vi "Build Help.vi"(8 "Error In":errorcluster) -> (0 "Error Out":errorcluster, 3 "stdout":string)   [LabVIEW 2017, in "Scripts.lvlib"]
uses:
  Scripts.lvlib
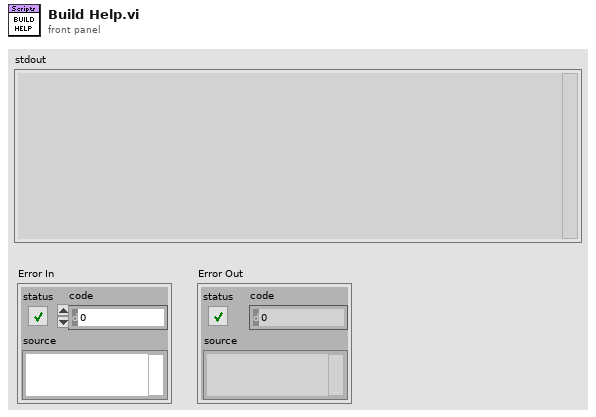
[diagram p1: front panel]
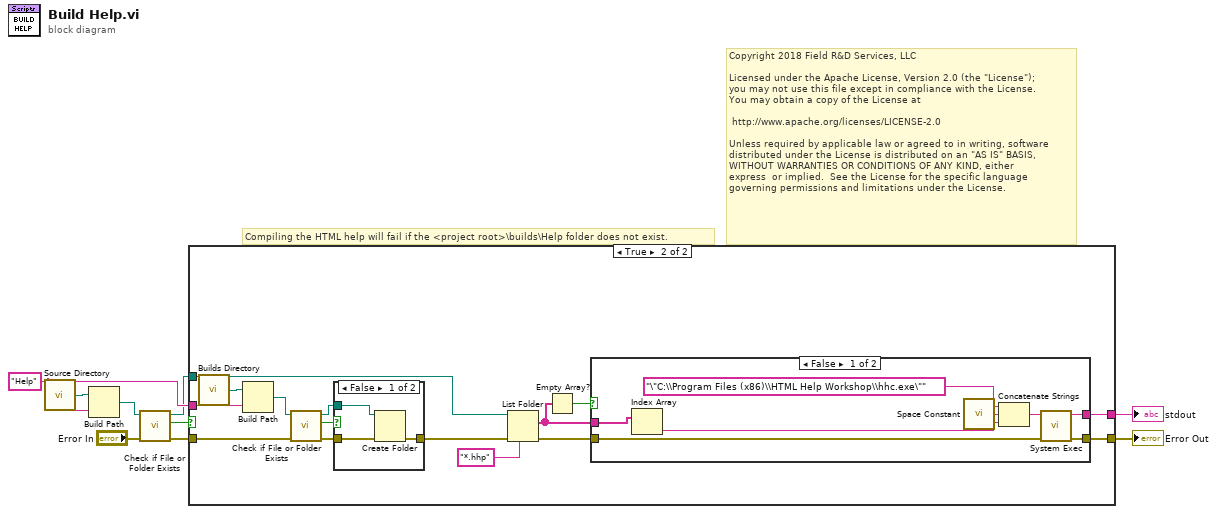
[diagram p0: block diagram]
diagram:
  w5 = "Help" ("name or relative path")
  # "Copyright 2018 Field R&D Services, LLC\n\nLicensed under the Apache License, Version 2.0 (the \"License\");\nyou may not use this file except in compliance with the License.\nYou may obtain a copy of the License at\n\n\thttp://www.apache.org/licenses/LICENSE-2.0\n\nUnless required by applicable law or agreed to in writing, software\ndistributed under the License is distributed on an \"AS IS\" BASIS,\nWITHOUT WARRANTIES OR CONDITIONS OF ANY KIND, either \nexpress  or implied.  See the License for the specific language \ngoverning permissions and limitations under the License."
  # "Compiling the HTML help will fail if the <project root>\\builds\\Help folder does not exist."
  n1 = call "Source Directory.vi"() -> ("Source Directory"=w9:path)
  n2 = Build Path(base path=w9, name or relative path=w5) -> (appended path=w6:path)
  n3 = call <vilib>:"Check if File or Folder Exists.vi"("error in (no error)"="Error In", "path"=w6) -> ("error out"=w1:errorcluster, "file or folder exists?"=w3:bool, "dup path"=w4:path)  [unwired: 7 in]
  n4 = case shown="True" w3 {
    tunnel: [w10 w25] -> w8
    tunnel: [_ w24] -> w7
    tunnel: w4 -> [_ w19]
    tunnel: w5 -> [_ w17]
    tunnel: w1 -> [w10 w16]
    frame False {
    }
    frame True {
      n5 = call "Builds Directory.vi"() -> ("Builds Directory"=w18:path)
      n6 = Build Path(base path=w18, name or relative path=w17) -> (appended path=w15:path)
      n7 = call <vilib>:"Check if File or Folder Exists.vi"("error in (no error)"=w16, "path"=w15) -> ("error out"=w13:errorcluster, "file or folder exists?"=w11:bool, "dup path"=w14:path)  [unwired: 7 in]
      n8 = case shown="False" w11 {
        tunnel: w14 -> [w28 _]
        tunnel: w13 -> [w27 w29]
        tunnel: [w26 w29] -> w12
        frame False {
          n9 = Create Folder(path (use dialog)=w28, error in=w27) -> (error out=w26:errorcluster)  [unwired: 1 in, 2 out]
        }
        frame True {
        }
      }
      n10 = List Folder(path=w19, pattern="*.hhp", error in=w12) -> (filenames=w20:string[], error out=w21:errorcluster)  [unwired: 1 in, 2 out]
      n11 = Empty Array?(array=w20) -> (empty?=w22:bool)
      n12 = case shown="False" w22 {
        tunnel: [w37 w38] -> w25
        tunnel: [w36 _] -> w24
        tunnel: w21 -> [w30 w38]
        tunnel: w20 -> [w32 _]
        frame False {
          n13 = Index Array(array=w32) -> (element=w31:string)  [unwired: 1 in]
          n14 = call <vilib>:"Space Constant.vi"() -> ("String"=w34:string)
          n15 = Concatenate Strings("\"C:\\Program Files (x86)\\HTML Help Workshop\\hhc.exe\"", w34, w31) -> (w33:string)
          n16 = call <vilib>:"System Exec.vi"("error in (no error)"=w30, "command line"=w33) -> ("error out"=w37:errorcluster, "standard output"=w36:string)  [unwired: 6 in, 2 out]
        }
        frame True {
        }
      }
    }
  }
  "Error Out" <- w8
  "stdout" <- w7
